vi "UMB_WallFollow.vi"(8 "behavior weights":i8[](array[numeric]), 10 "tweakers cluster":T1, 11 "ir distance":i32) -> (3 "Behavior Output":T2)   [LabVIEW 2012]
uses:
  NINJA Code/Tugboat/Robo_Programs/behaviorOutput_t.ctl
  <vilib>/gmath/statdist.llb/Normal PDF.vi
  <vilib>/gmath/NI_Gmath.lvlib
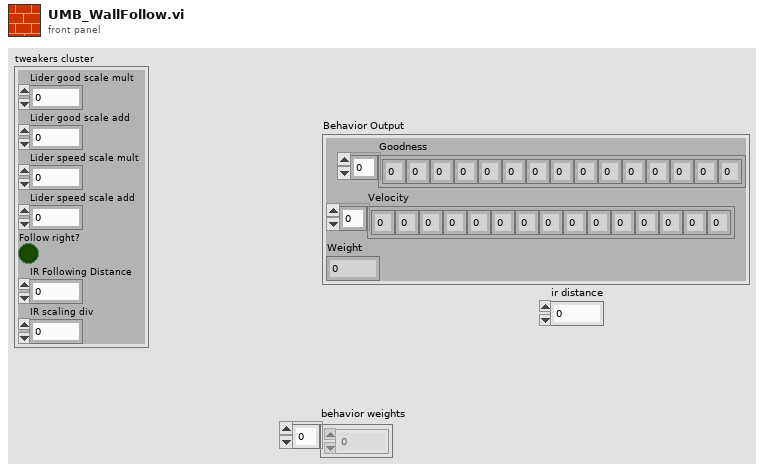
[diagram p1: front panel]
types:
  T1 = cluster{"Lider good scale mult":i32, "Lider good scale add":i32, "Lider speed scale mult":i32, "Lider speed scale add":i32, "Follow right?":bool, "IR Following Distance":i32, "IR scaling div":i32}
  T2 = typedef "behaviorOutput_t.ctl" = cluster{"Goodness":i8[], "Velocity":i8[], "Weight":i8}
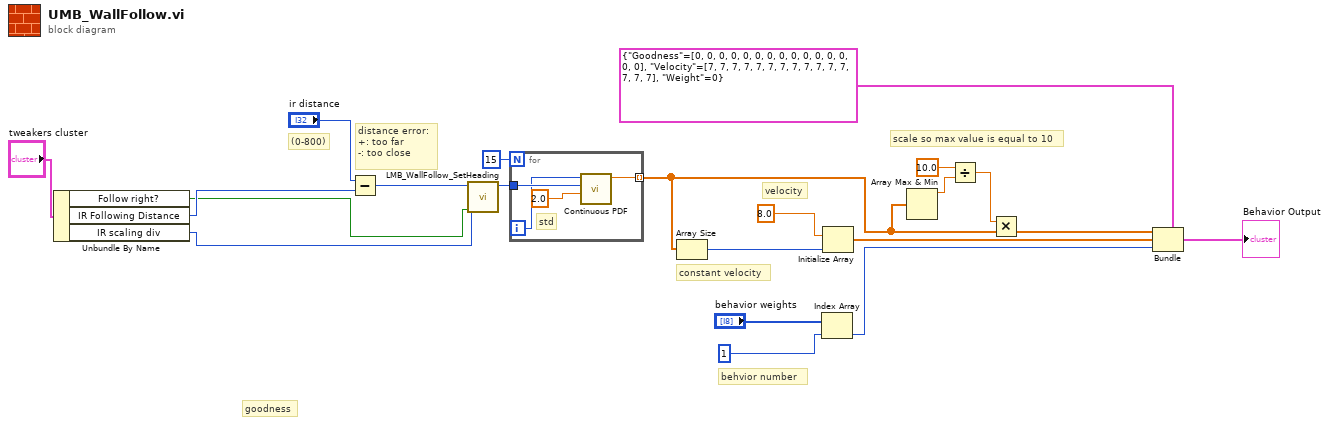
[diagram p0: block diagram]
diagram:
  # "scale so max value is equal to 10"
  # "(0-800)"
  # "constant velocity"
  # "velocity"
  # "goodness"
  # "distance error: \n+: too far\n-: too close"
  # "behvior number"
  n1 = Unbundle By Name("tweakers cluster") -> ("Follow right?"=w1:bool, "IR Following Distance"=w2:i32, "IR scaling div"=w3:i32)
  n2 = Subtract(x="ir distance", y=w2) -> (x-y=w15:i32)
  n3 = call "LMB_WallFollow_SetHeading.vi"("Follow Right?"=w1, "division constant"=w3, "Distance error"=w15) -> ("heading"=w14:i32)  [unwired: 8 in]
  n4 = for {
    N: 15 -> [_]
    tunnel: w14 -> [w25]
    tunnel: [w23] -> w5 mode=indexing
    i -> [w22]
    # "std"
    n5 = call-poly <vilib>:"Continuous PDF.vi"("std"=2.0, "mean"=w25, "x"=w22) -> ("pdf(x)"=w23:dbl)  [unwired: 7 in, 1 out]
  }
  n6 = Array Size(array=w5) -> (size(s)=w11:i32)
  n7 = Index Array(array="behavior weights", index=1) -> (element=w19:i8)
  n8 = Initialize Array(8.0 ("element"), w11) -> (w12:dbl[])
  n9 = Array Max & Min(array=w5) -> (max value=w7:dbl)  [unwired: 3 out]
  n10 = Divide(x=10.0, y=w7) -> (x/y=w6:dbl)
  n11 = Multiply(x=w6, y=w5) -> (x*y=w9:dbl[])
  n12 = Bundle(cluster=T2 {"Goodness"=[0, 0, 0, 0, 0, 0, 0, 0, 0, 0, 0, 0, 0, 0, 0], "Velocity"=[7, 7, 7, 7, 7, 7, 7, 7, 7, 7, 7, 7, 7, 7, 7], "Weight"=0} ("Behavior Output"), "Goodness"=w9, "Velocity"=w12, "Weight"=w19) -> (→"Behavior Output":T2)
